vi "Sync.vi"(8 "error in (no error)":errorcluster, 10 "timeout in ms (-1)":i32, 11 "Abs_Sync in":refnum<class "Abs_Sync.lvclass">) -> (0 "error out":errorcluster, 2 "timed out?":bool, 3 "Abs_Sync out":refnum<class "Abs_Sync.lvclass">)   [LabVIEW 2019, in "Abs_Sync.lvclass"]
uses:
  LV_Abstract/Source/Abs_Types/Interfaces/Sync/Abs_Sync.lvclass
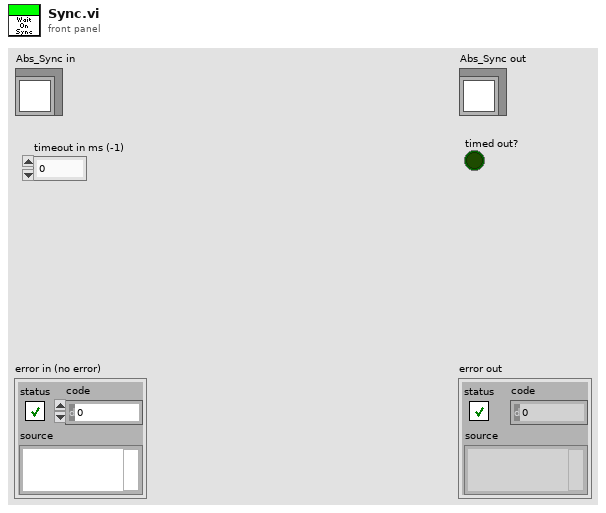
[diagram p1: front panel]
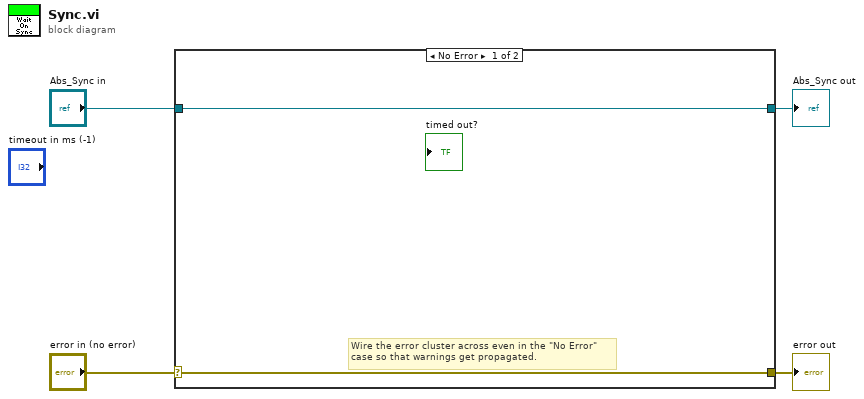
[diagram p0: block diagram]
diagram:
  n1 = case shown="No Error" "error in (no error)" {
    selector: "error in (no error)" -> [w5 w8]
    tunnel: [w5 w8] -> w3
    tunnel: [w6 w7] -> w1
    tunnel: "Abs_Sync in" -> [w6 w7]
    frame No Error {
      # "Wire the error cluster across even in the \"No Error\"\ncase so that warnings get propagated."
    }
    frame Error {
    }
  }
  "error out" <- w3
  "Abs_Sync out" <- w1
